vi "Check Window Bounds.vi"(8 "error in":errorcluster, 11 "File Info in":T1) -> (0 "error out":errorcluster, 3 "File Info out":T1)   [LabVIEW 2020, in "Peer Review.lvclass"]
uses:
  Peer Review.lvclass
  TypeDefs/File Info.ctl
  TypeDefs/File State.ctl
  TypeDefs/VI Type.ctl
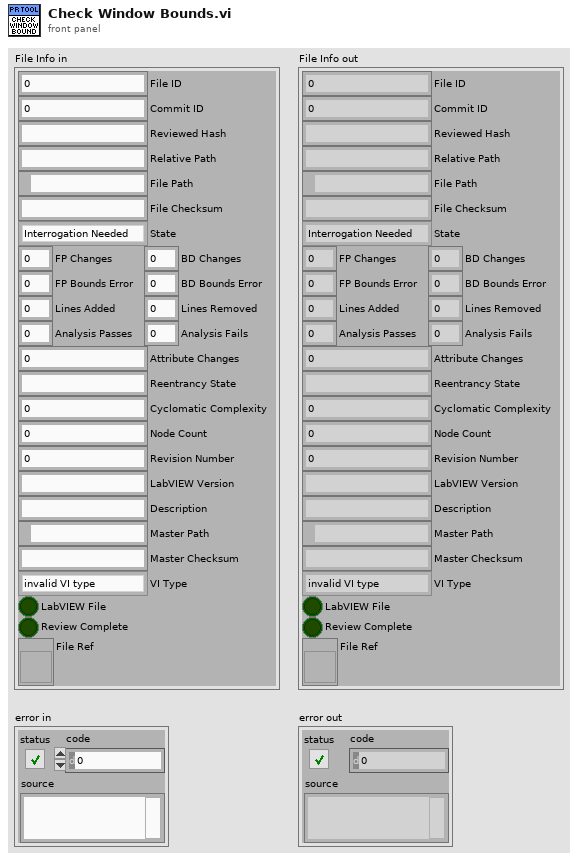
[diagram p1: front panel]
types:
  T1 = typedef "Peer Review.lvclass/File Info.ctl" = cluster{"File ID":i32, "Commit ID":i32, "Reviewed Hash":string, "Relative Path":string, "File Path":path, "File Checksum":string, "State":T2, "FP Changes":i32, "BD Changes":i32, "FP Bounds Error":dbl, "BD Bounds Error":dbl, "Lines Added":i32, "Lines Removed":i32, "Analysis Passes":i32, "Analysis Fails":i32, "Attribute Changes":i32, "Reentrancy State":string, "Cyclomatic Complexity":i32, "Node Count":i32, "Revision Number":u32, "LabVIEW Version":string, "Description":string, "Master Path":path, "Master Checksum":string, "VI Type":T3, "LabVIEW File":bool, "Review Complete":bool, "File Ref":refnum<vi>}
  T2 = typedef "Peer Review.lvclass/File State.ctl" = enum16{"Interrogation Needed", "Modified", "Deleted", "Added", "Matches Previous", "No Changes", "Moved"}
  T3 = typedef "Peer Review.lvclass/VI Type.ctl" = enum32{"invalid VI type", "Standard VI", "Control VI", "Global VI", "Polymorphic VI", "Configuration VI", "SubSystem", "Facade VI", "Method VI", "Statechart Diagram VI"}
  T4 = typedef "LVRectTypeDef.ctl" = cluster{"Left":i16, "Top":i16, "Right":i16, "Bottom":i16}
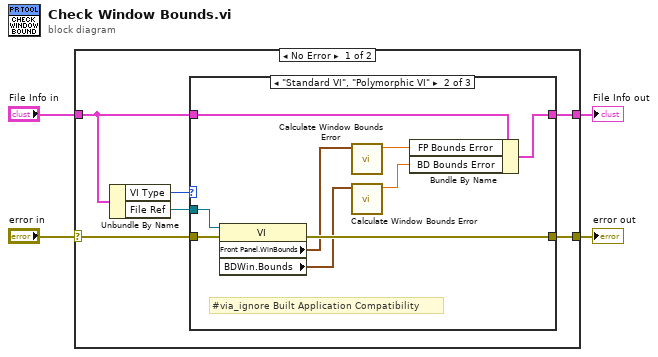
[diagram p0: block diagram]
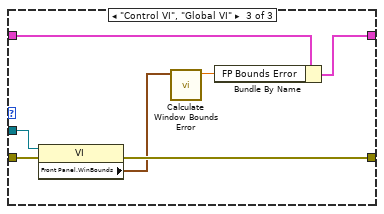
[diagram p3: hidden frame]
diagram:
  n1 = case shown="No Error" "error in" {
    selector: "error in" -> [w6 w30]
    tunnel: [w10 w30] -> w4
    tunnel: "File Info in" -> [w9 w29]
    tunnel: [w8 w29] -> w1
    frame No Error {
      n2 = Unbundle By Name(w9) -> ("VI Type"=w7:T3, "File Ref"=w5:refnum<vi>)
      n3 = case shown="\"Standard VI\", \"Polymorphic VI\"" w7 {
        tunnel: [w12 w19 w26] -> w10
        tunnel: w6 -> [w12 w20 w27]
        tunnel: w5 -> [_ w21 w28]
        tunnel: w9 -> [w11 w17 w23]
        tunnel: [w11 w15 w22] -> w8
        frame Default {
        }
        frame "Standard VI", "Polymorphic VI" {
          # "#via_ignore Built Application Compatibility"
          n4 = property on="Property Node" class="VI"(reference=w21, error in=w20) -> (error out=w19:errorcluster, "Front Panel.WinBounds"=w18:T4, "BDWin.Bounds"=w14:T4)  [unwired: 1 out]
          n5 = call "Calculate Window Bounds Error.vi"("Window Bounds"=w18) -> ("Error (%)"=w16:dbl)  [unwired: 10 in]
          n6 = call "Calculate Window Bounds Error.vi"("Window Bounds"=w14) -> ("Error (%)"=w13:dbl)  [unwired: 10 in]
          n7 = Bundle By Name(cluster=w17, "FP Bounds Error"=w16, "BD Bounds Error"=w13) -> (w15:T1)
        }
        frame "Control VI", "Global VI" {
          n8 = property on="Property Node" class="VI"(reference=w28, error in=w27) -> (error out=w26:errorcluster, "Front Panel.WinBounds"=w24:T4)  [unwired: 1 out]
          n9 = call "Calculate Window Bounds Error.vi"("Window Bounds"=w24) -> ("Error (%)"=w25:dbl)  [unwired: 10 in]
          n10 = Bundle By Name(cluster=w23, "FP Bounds Error"=w25) -> (w22:T1)
        }
      }
    }
    frame Error {
    }
  }
  "error out" <- w4
  "File Info out" <- w1
